vi "LEDStripSet.vi"(8 "error in":errorcluster, 10 "Color":u32, 11 "LEDStripRef in":T1={"PWM Rate (Hz)"=1000.0, "Max Duty Cycle"=0.0, "DigitalOutputRed"={"Digital Module"=enum."Digital Module 1", "DIO Channel"=enum."DIO 1", "DevStatus"={"status"=FALSE, "code"=0, "source"=""}}, "DigitalOutputGreen"={"Digital Module"=enum."Digital Module 1", "DIO Channel"=enum."DIO 1", "DevStatus"={"status"=FALSE, "code"=0, "source"=""}}, "DigitalOutputBlue"={"Digital Module"=enum."Digital Module 1", "DIO Channel"=enum."DIO 1", "DevStatus"={"status"=FALSE, "code"=0, "source"=""}}, "DevStatus"={"status"=FALSE, "code"=0, "source"=""}}) -> (0 "error out":errorcluster, 3 "LEDStripRef out":T1={"PWM Rate (Hz)"=1000.0, "Max Duty Cycle"=0.0, "DigitalOutputRed"={"Digital Module"=enum."Digital Module 1", "DIO Channel"=enum."DIO 1", "DevStatus"={"status"=FALSE, "code"=0, "source"=""}}, "DigitalOutputGreen"={"Digital Module"=enum."Digital Module 1", "DIO Channel"=enum."DIO 1", "DevStatus"={"status"=FALSE, "code"=0, "source"=""}}, "DigitalOutputBlue"={"Digital Module"=enum."Digital Module 1", "DIO Channel"=enum."DIO 1", "DevStatus"={"status"=FALSE, "code"=0, "source"=""}}, "DevStatus"={"status"=FALSE, "code"=0, "source"=""}})   [LabVIEW 2014]
uses:
  LEDStripRef.ctl
  <vilib>/Rock Robotics/WPI/DigitalOutput/WPI_DigitalOutputDevRef.ctl
  <vilib>/Rock Robotics/SystemInterfaces/Typedef/FPGA_TypedefDigitalModule.ctl
  <vilib>/Rock Robotics/SystemInterfaces/DIO/FPGA_DIOChannel.ctl
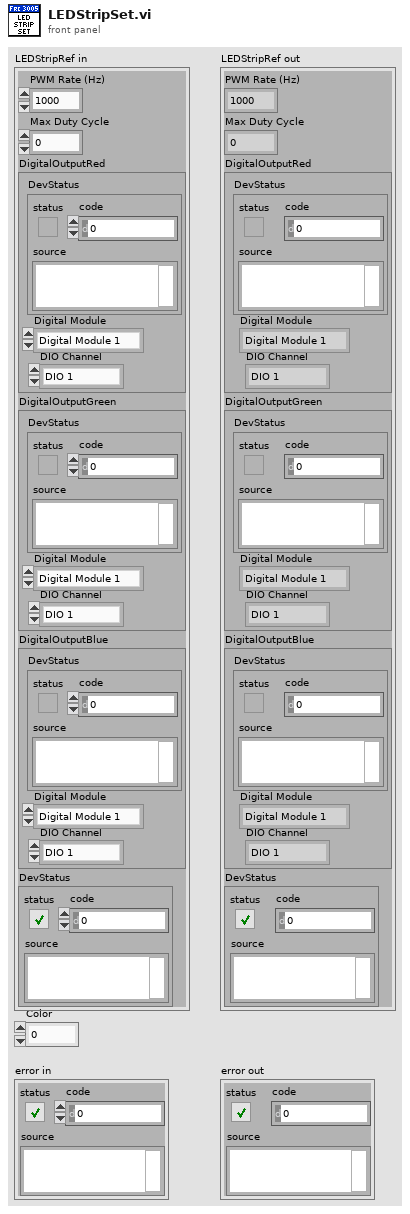
[diagram p1: front panel]
types:
  T1 = typedef "LEDStripRef.ctl" = cluster{"PWM Rate (Hz)":sgl, "Max Duty Cycle":sgl, "DigitalOutputRed":T2, "DigitalOutputGreen":T2, "DigitalOutputBlue":T2, "DevStatus":errorcluster}
  T2 = typedef "WPI_DigitalOutputDevRef.ctl" = cluster{"Digital Module":T3, "DIO Channel":T4, "DevStatus":errorcluster}
  T3 = typedef "FPGA_TypedefDigitalModule.ctl" = enum16{"Digital Module 1", "Digital Module 2"}
  T4 = typedef "FPGA_DIOChannel.ctl" = enum8{"DIO 1", "DIO 2", "DIO 3", "DIO 4", "DIO 5", "DIO 6", "DIO 7", "DIO 8", "DIO 9", "DIO 10", "DIO 11", "DIO 12", "DIO 13", "DIO 14", "Invalid"}
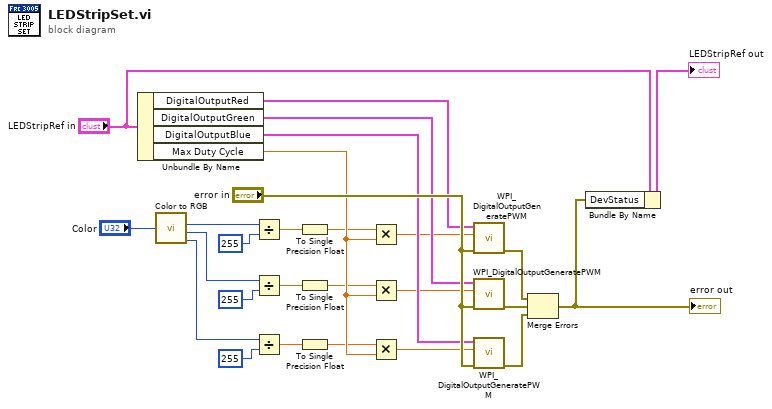
[diagram p0: block diagram]
diagram:
  n1 = Unbundle By Name("LEDStripRef in") -> ("DigitalOutputRed"=w16:T2, "DigitalOutputGreen"=w15:T2, "DigitalOutputBlue"=w14:T2, "Max Duty Cycle"=w4:sgl)
  n2 = call <vilib>:"Color to RGB.vi"("Color"="Color") -> ("R"=w21:u8, "G"=w18:u8, "B"=w17:u8)  [unwired: 1 out]
  n3 = Divide(x=w21, y=u8 255 ("R")) -> (x/y=w10:dbl)
  n4 = Divide(x=w18, y=u8 255 ("R")) -> (x/y=w9:dbl)
  n5 = Divide(x=w17, y=u8 255 ("R")) -> (x/y=w8:dbl)
  n6 = To Single Precision Float(number=w10) -> (single precision float=w1:sgl)
  n7 = To Single Precision Float(number=w9) -> (single precision float=w2:sgl)
  n8 = To Single Precision Float(number=w8) -> (single precision float=w3:sgl)
  n9 = Multiply(x=w1, y=w4) -> (x*y=w7:sgl)
  n10 = Multiply(x=w2, y=w4) -> (x*y=w6:sgl)
  n11 = Multiply(x=w3, y=w4) -> (x*y=w5:sgl)
  n12 = call <vilib>:"WPI_DigitalOutputGeneratePWM.vi"("error in (no error)"="error in", "PWM Duty Cycle"=w7, "DigitalOutputDevRef"=w16) -> ("error out"=w11:errorcluster)  [unwired: 7 in, 1 out]
  n13 = call <vilib>:"WPI_DigitalOutputGeneratePWM.vi"("error in (no error)"="error in", "PWM Duty Cycle"=w6, "DigitalOutputDevRef"=w15) -> ("error out"=w12:errorcluster)  [unwired: 7 in, 1 out]
  n14 = call <vilib>:"WPI_DigitalOutputGeneratePWM.vi"("error in (no error)"="error in", "PWM Duty Cycle"=w5, "DigitalOutputDevRef"=w14) -> ("error out"=w13:errorcluster)  [unwired: 7 in, 1 out]
  n15 = Merge Errors(w11, w12, w13) -> (w26:errorcluster)
  "error out" <- w26
  n16 = Bundle By Name(cluster="LEDStripRef in", "DevStatus"=w26) -> (→"LEDStripRef out":T1)
